vi "Initialize Compass.vi"(8 "error in (no error)":errorcluster, 11 "Device ID":T1) -> (0 "error out":errorcluster, 2 "Sensor Error":i32, 3 "Honeywell Compass HMC6343":refnum<class "Honeywell Compass HMC6343.lvclass">)   [LabVIEW 2012, in "UniCyRO.lvlib" / "UniCyRO_Host_Sim.lvclass"]
uses:
  UniCyRO_Host_Sim.lvclass
  <vilib>/robotics/Simulator/Engine/ctl/DeviceID.ctl
  <instrlib>/Honeywell Compass HMC6343/HAIOL/Honeywell Compass HMC6343.lvclass
  <vilib>/robotics/Utilities/NI_Robotics Utilities.lvlib
  <instrlib>/Honeywell Compass HMC6343/HAIOL/Simulator/Honeywell Compass HMC6343 Simulator.lvclass
  <vilib>/robotics/Simulator/NI_Robotics_Simulator.lvlib
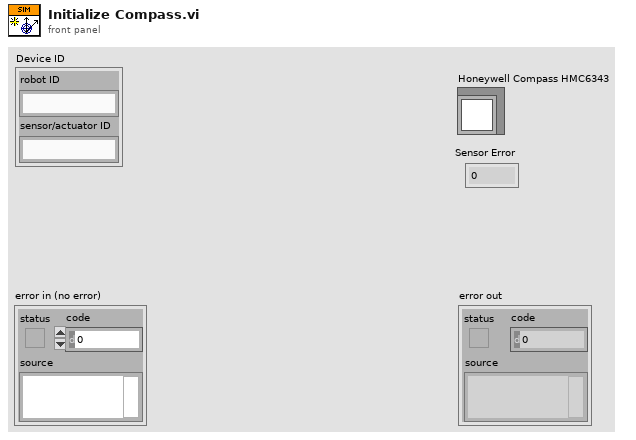
[diagram p1: front panel]
types:
  T1 = typedef "NI_Robotics_Simulator.lvlib/DeviceID.ctl" = cluster{"robot ID":string, "sensor/actuator ID":string}
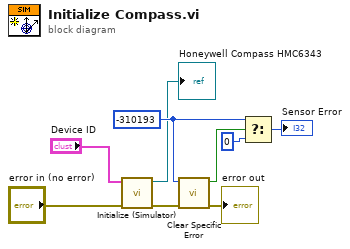
[diagram p0: block diagram]
diagram:
  w6 = -310193 ("code")
  n1 = call <instrlib>:"Initialize (Simulator).vi"("error in (no error)"="error in (no error)", "Device ID"="Device ID") -> ("error out"=w1:errorcluster, "Honeywell Compass HMC6343"=→"Honeywell Compass HMC6343":refnum<class "Honeywell Compass HMC6343.lvclass">)  [unwired: 8 in]
  n2 = call <vilib>:"Clear Specific Error.vi"("error in (no error)"=w1, "code"=w6) -> ("error out"=→"error out":errorcluster, "code found?"=w7:bool)  [unwired: 7 in, 1 out]
  n3 = Select(t=w6, s=w7, f=0) -> (s? t:f=→"Sensor Error":i32)
